vi "SiosIfmSetMeasurement.vi"(1 "OutputWordRate":dbl, 2 "measurementFlag":u32, 3 "int32DeviceNumber":i32) -> (0 "success":i32)   [LabVIEW 2009]
uses:
  siosifm.dll
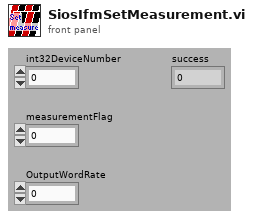
[diagram p1: front panel]
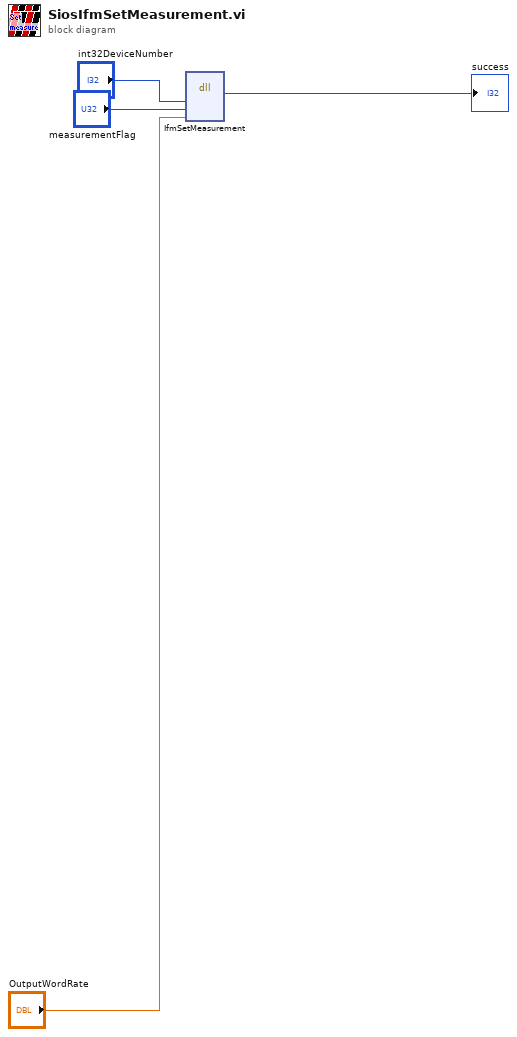
[diagram p0: block diagram]
diagram:
  n1 = dll-call lib="D:/Support/Labview/RE-10/SIOS_IfmDLL/siosifm.dll" fn="IfmSetMeasurement"("deviceNumber"="int32DeviceNumber", "measurementFlags"="measurementFlag", "outputWordRate"="OutputWordRate") -> (→"success":i32)  [unwired: 6 in, 2 out]
